vi "0_set_default_parameters.vi"(10 "1 width (ns)":dbl=14.0, 11 "Pulse Generator":bool) -> ()   [LabVIEW 2013]
panel:
  in  "Keysight Connection":T1={"Type"=1, "VISA"="TCPIP0::192.168.0.8::inst0::INSTR", "GPIB"="10"} {"Type" items=["VISA", "GPIB"]}
  in  "Outputs":T2={"Ouput 1"=TRUE, "Ouput 2"=TRUE, "Ouput 1 Neg"=TRUE, "Ouput 2 Neg"=TRUE}
  in  "Frequency Parameters":T3={"Coupling"=FALSE, "Frequency 2 (MHz)"=2.0, "Frequency 1 (MHz)"=3.0, "WAVEFORM"=enum."ARBITRARY"} {"Frequency 1 (MHz)" min=0.0 max=14.5; "Frequency 2 (MHz)" min=0.0 max=14.5}
  in  "Yokogawa Address":refnum<visa-resource-name>="USB0::0x0B21::0x0039::91NA15589::INSTR"
  in  "Generator Output":bool
  in  "Power  (dBm)":dbl=10.0
  in  "Frequency (Hz)":dbl=6953330000.0 format="%#_10p"
  in  "Generator":bool
  in  "Current":bool
  in  "VNA":bool
  in  "I mA":dbl=-0.176 step=2e-05
  in  "Center Freq (Hz)":dbl=8583250000.0 format="%#.6p"
  in  "Power dBm":dbl=-5.0 caption="Power (dBm)" format="%#.3f"
  in  "2 delay (ns)":dbl
  in  "1 delay (ns)":dbl
  in  "2 width (ns)":dbl=20.0
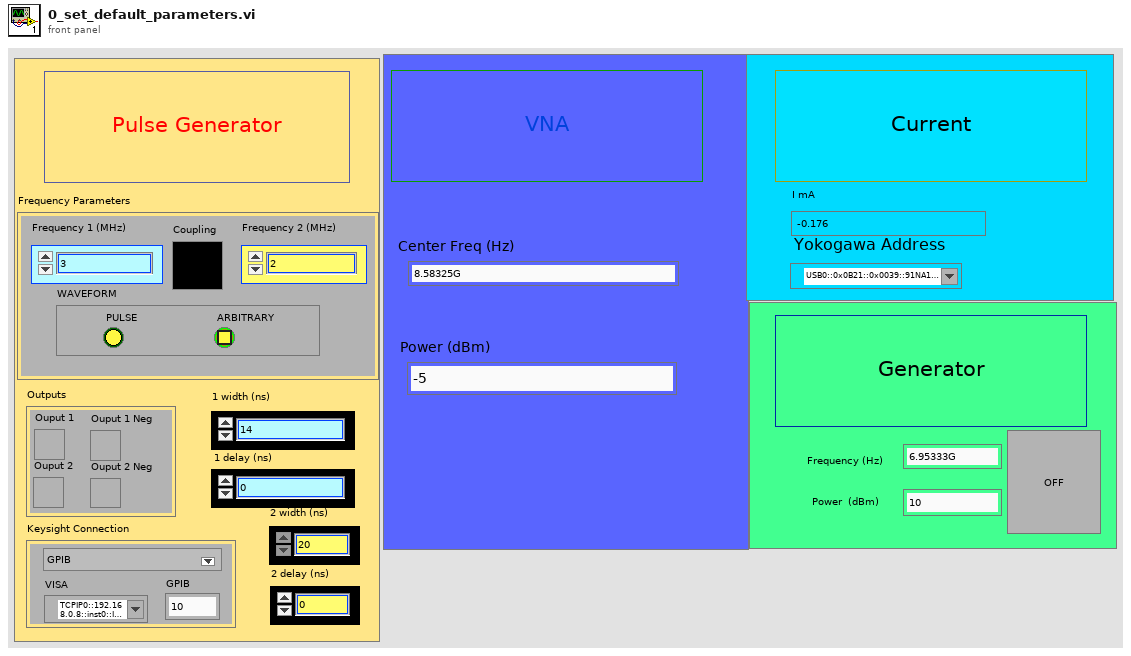
[diagram p1: front panel]
types:
  T1 = cluster{"Type":u16, "VISA":refnum<visa-resource-name>, "GPIB":string}
  T2 = cluster{"Ouput 1":bool, "Ouput 2":bool, "Ouput 1 Neg":bool, "Ouput 2 Neg":bool}
  T3 = cluster{"Coupling":bool, "Frequency 2 (MHz)":dbl, "Frequency 1 (MHz)":dbl, "WAVEFORM":enum32{"PULSE", "ARBITRARY"}}
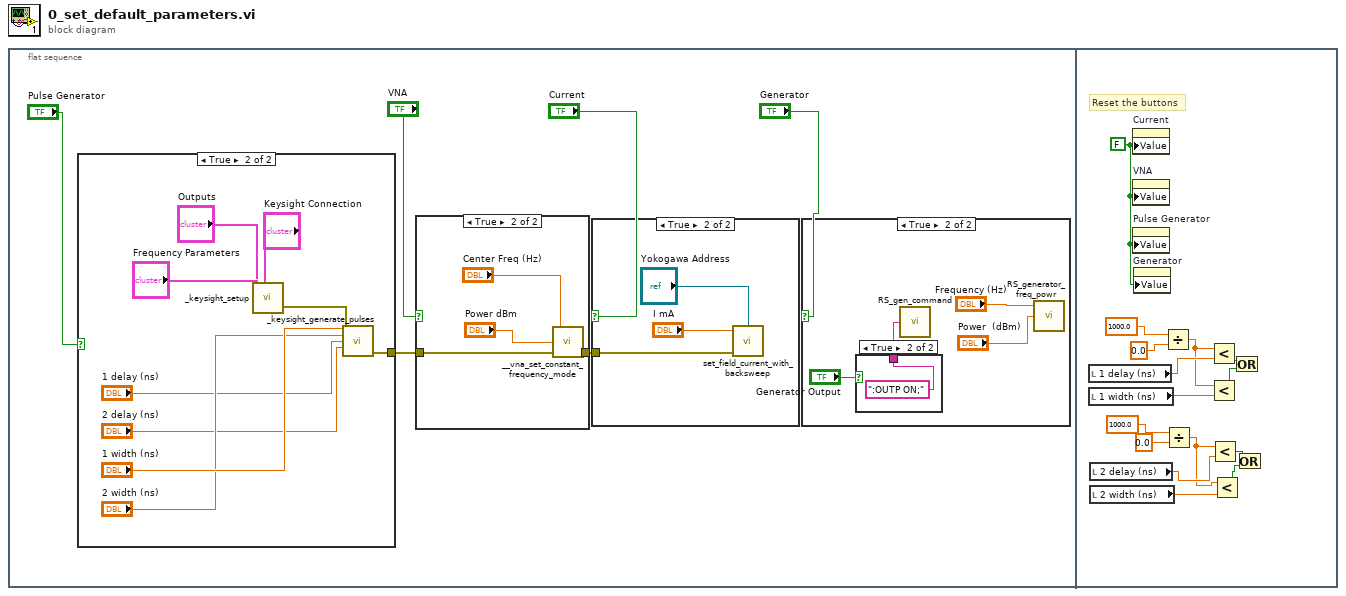
[diagram p0: block diagram]
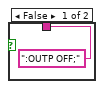
[diagram p3: hidden frame]
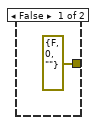
[diagram p6: hidden frame]
diagram:
  n1 = flat-sequence {
    frame #0 {
      n2 = case shown="True" "Pulse Generator" {
        tunnel: [errorcluster {"status"=FALSE, "code"=0, "source"=""} ("error out") w25] -> w6
        frame False {
        }
        frame True {
          n3 = call "_keysight_setup.vi"("Frequency Parameters"="Frequency Parameters", "Outputs"="Outputs", "Keysight Connection"="Keysight Connection") -> ("error out"=w30:errorcluster)  [unwired: 3 in]
          n4 = call "_keysight_generate_pulses.vi"("Ch1 pulse_width (ns)"="1 width (ns)", "Ch2 pulse_width (ns)"="2 width (ns)", "Ch1 pulse_delay (ns)"="1 delay (ns)", "Ch2 pulse_delay (ns)"="2 delay (ns)", "error in"=w30) -> ("error out"=w25:errorcluster)  [unwired: 9 in, 1 out]
        }
      }
      n5 = case shown="True" "VNA" {
        tunnel: w6 -> [w16 w20]
        tunnel: [w16 w19] -> w5
        frame False {
        }
        frame True {
          n6 = call "__vna_set_constant_frequency_mode.vi"("error in (no error)"=w20, "Power dBm"="Power dBm", "Center Freq (Hz):"="Center Freq (Hz)") -> ("error out"=w19:errorcluster)  [unwired: 2 in]
        }
      }
      n7 = case shown="True" "Current" {
        tunnel: w5 -> [_ w15]
        frame False {
        }
        frame True {
          n8 = call "set_field_current_with_backsweep.vi"("Yokogawa Address"="Yokogawa Address", "error in"=w15, "I mA"="I mA") -> ()  [unwired: 2 in, 1 out]
        }
      }
      n9 = case shown="True" "Generator" {
        frame False {
        }
        frame True {
          n10 = case shown="True" "Generator Output" {
            tunnel: [":OUTP OFF;" ":OUTP ON;"] -> w9
            frame False {
            }
            frame True {
            }
          }
          n11 = call "RS_gen_command.vi"("Comand"=w9) -> ()  [unwired: 4 in, 1 out]
          n12 = call "RS_generator_freq_powr.vi"("Power (dBm)"="Power  (dBm)", "Frequnecy (Hz)"="Frequency (Hz)") -> ()  [unwired: 1 in, 2 out]
        }
      }
    }
    frame #1 {
      w33 = FALSE ("Current")
      # "Reset the buttons"
      n13 = local read "1 delay (ns)"() -> (w43:dbl)
      n14 = local read "1 width (ns)"() -> (w39:dbl)
      n15 = local read "2 delay (ns)"() -> (w38:dbl)
      n16 = local read "2 width (ns)"() -> (w37:dbl)
      n17 = property on="Current" class="Bool (strict)"("Value"=w33) -> ()  [unwired: 2 in, 2 out]
      n18 = property on="VNA" class="Bool (strict)"("Value"=w33) -> ()  [unwired: 2 in, 2 out]
      n19 = property on="Pulse Generator" class="Bool (strict)"("Value"=w33) -> ()  [unwired: 2 in, 2 out]
      n20 = property on="Generator" class="Bool (strict)"("Value"=w33) -> ()  [unwired: 2 in, 2 out]
      n21 = Divide(x=1000.0, y=0.0) -> (x/y=w40:dbl)
      n22 = Divide(x=1000.0, y=0.0) -> (x/y=w36:dbl)
      n23 = Less?(x=w40, y=w43) -> (x < y?=w41:bool)
      n24 = Less?(x=w40, y=w39) -> (x < y?=w42:bool)
      n25 = Less?(x=w36, y=w38) -> (x < y?=w34:bool)
      n26 = Less?(x=w36, y=w37) -> (x < y?=w35:bool)
      n27 = Or(x=w41, y=w42) -> ()  [unwired: 1 out]
      n28 = Or(x=w34, y=w35) -> ()  [unwired: 1 out]
    }
  }
